vi "Connect and init controller.vi"(7 "axis (0)":u32(ring) items=["1", "2", "3"], 8 "error in (no error)":errorcluster, 9 "Interface types":u32(ring)=1 items=["None", "USB", "TCP", "All"], 10 "path to LUT":path, 11 "path to dll":path) -> (0 "error out":errorcluster, 2 "Rotator":T1={"Controller info"={"deviceNumber"=0, "DeviceType"=3, "ID"=0, "Serial"="", "Address"="", "connected"=FALSE}, "Handle"=0, "FW-Version"=0, "Features"=0, "ActuatorType"=0, "ActuatorName"="", "Axis info"={"Axis status"={"connected"=FALSE, "enabled"=FALSE, "moving"=FALSE, "target"=FALSE, "EotFwd"=FALSE, "EotBwd"=FALSE, "error"=FALSE}, "Position [°]"=0.0, "Freque [Hz]"=0.0, "Voltage [V]"=0.0}, "Capacitance[uF]"=0.0, "Path to DLL"=path ""} {"ActuatorType" items=["Linear", "Rotator", "Goniometer"]; "Controller info"."DeviceType" items=["ANC350res", "ANC350num", "ANC350fps", "No device / invalid"]; "Controller info"."ID" format="%x"})   [LabVIEW 2024, in "SampleRotator.lvlib"]
doc: "Searches for ANC350 devices connected by USB. Connects to first one and reads its info.\n\ninputs:\nPath to DLL; error cluster.\n\noutputs:\nANC350_handle; Controller info; number of found devices; error cluster."
uses:
  SampleRotator.lvlib
  ctl/Rotator all.ctl
  ctl/Axis status.ctl
  <vilib>/Utility/error.llb/Error Cluster From Error Code.vi
  <vilib>/ErrorRing/Error Ring.xnode
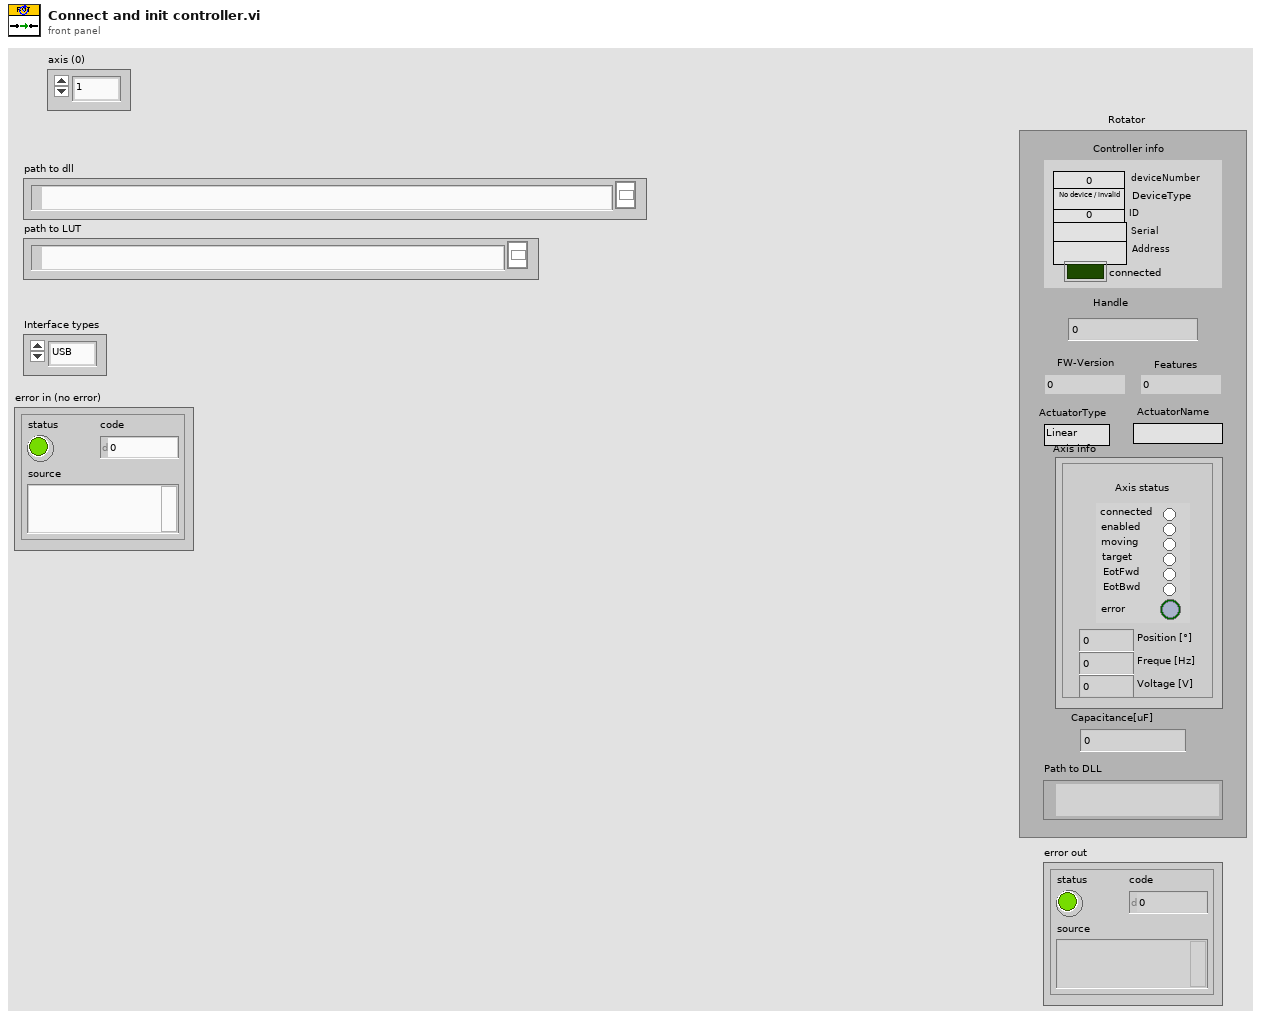
[diagram p1: front panel]
types:
  T1 = typedef "SampleRotator.lvlib/Rotator all.ctl" = cluster{"Controller info":cluster{"deviceNumber":i32, "DeviceType":i32, "ID":u32, "Serial":string, "Address":string, "connected":bool}, "Handle":u64, "FW-Version":i32, "Features":u32, "ActuatorType":u16, "ActuatorName":string, "Axis info":T2, "Capacitance[uF]":dbl, "Path to DLL":path}
  T2 = typedef "SampleRotator.lvlib/Axis status.ctl" = cluster{"Axis status":cluster{"connected":bool, "enabled":bool, "moving":bool, "target":bool, "EotFwd":bool, "EotBwd":bool, "error":bool}, "Position [°]":dbl, "Freque [Hz]":dbl, "Voltage [V]":dbl}
  T3 = cluster{"deviceNumber":i32, "DeviceType":i32, "ID":u32, "Serial":string, "Address":string, "connected":bool}
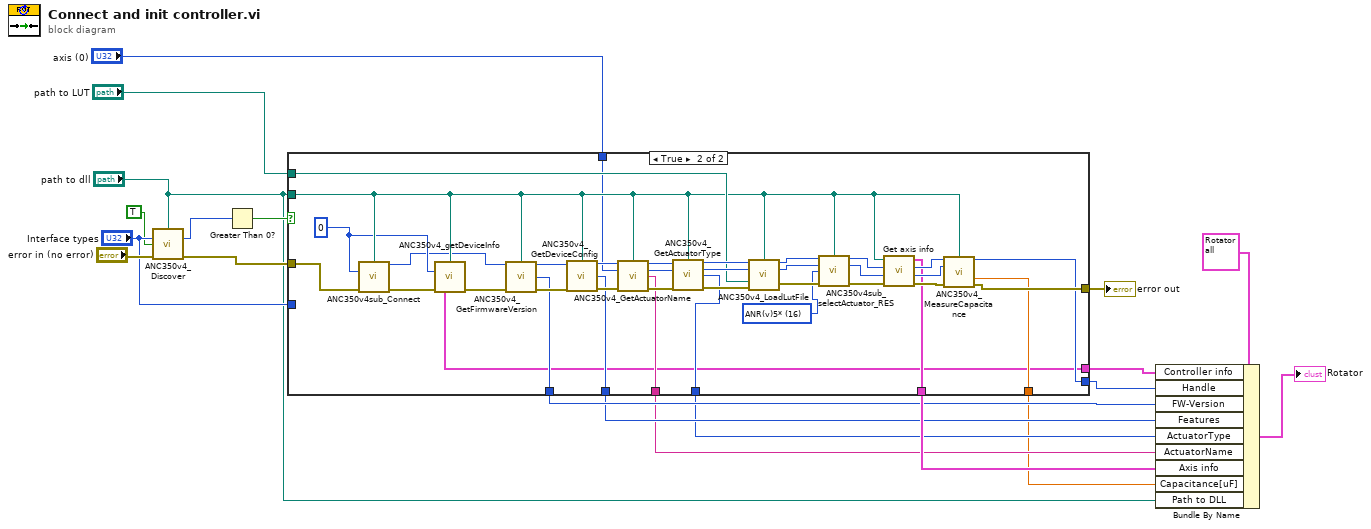
[diagram p0: block diagram]
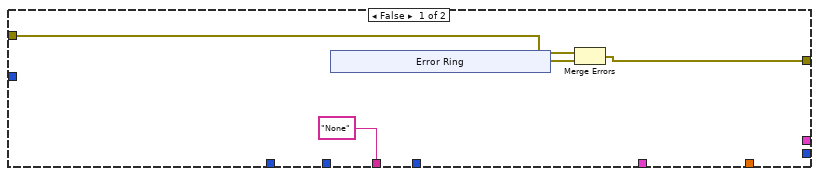
[diagram p2: hidden frame]
diagram:
  n1 = call <instrlib>:"ANC350v4_Discover.vi"("Path to *.DLL"="path to dll", "Interface types"="Interface types", "Load Library (T)\nUnload (F)"=TRUE ("Load Library (T)\nUnload (F)"), "error in"="error in (no error)") -> ("ANC350v4 found"=w16:u32, "error ANC350v4_discover"=w18:errorcluster)  [unwired: 10 in]
  n2 = Greater Than 0?(x=w16) -> (x > 0?=w17:bool)
  n3 = case shown="True" w17 {
    tunnel: "path to dll" -> [_ w33]
    tunnel: "Interface types" -> [_ _]
    tunnel: w18 -> [w22 w30]
    tunnel: [_ w34] -> w11
    tunnel: [w23 w44] -> w15
    tunnel: "path to LUT" -> [_ w57]
    tunnel: [_ w43] -> w10
    tunnel: [_ w42] -> w9
    tunnel: [_ w41] -> w8
    tunnel: [_ w40] -> w7
    tunnel: [_ w39] -> w6
    tunnel: ["None" ("ActuatorName") w38] -> w5
    tunnel: [_ w37] -> w4
    tunnel: "axis (0)" -> [_ w32]
    frame False {
      n4 = xnode "Error Ring"() -> ("error out"=w24:errorcluster)
      n5 = Merge Errors(w22, w24) -> (w23:errorcluster)
    }
    frame True {
      w31 = u32 0 ("deviceNumber")
      w53 = u16 16 items=["ANPx51"=0, "ANPz51"=1, "ANPz51ext"=2, "ANPx101"=3, "ANPz101"=4, "ANPz102"=5, "ANPz101ext"=6, "ANPz111(ext)"=7, "ANPx111(ext)"=8, "ANPx121"=9, "ANPx311"=10, "ANPx321"=11, "ANPx341"=12, "ANGt101"=13, "ANGp101"=14, "ANR(v)101"=15, "ANR(v)5*"=16, "ANR(v)200/240"=17, "ANR(v)220"=18, "Please select type"=99] ("RES-Positionierer")
      n6 = call <instrlib>:"ANC350v4sub_Connect.vi"("Path to *.DLL"=w33, "deviceNumber"=w31, "error in"=w30) -> ("ANC350v4_Handle_Out"=w29:u64, "error ANC350v4_Dis/Connect"=w36:errorcluster)  [unwired: 11 in]
      n7 = call <instrlib>:"ANC350v4_getDeviceInfo.vi"("Path to *.DLL"=w33, "deviceNumber"=w31, "error in"=w36) -> ("output cluster"=w34:T3, "Error_ANC350v4_getDeviceInfo"=w35:errorcluster)  [unwired: 5 in, 6 out]
      n8 = call <instrlib>:"ANC350v4_GetFirmwareVersion.vi"("deviceHandle"=w29, "Path to *.DLL"=w33, "error in"=w35) -> ("deviceHandle"=w51:u64, "FW-Version"=w41:i32, "error ANC350v4_getFirmwareVersion"=w52:errorcluster)  [unwired: 10 in]
      n9 = call <instrlib>:"ANC350v4_GetDeviceConfig.vi"("deviceHandle"=w51, "Path to *.DLL"=w33, "error in"=w52) -> ("deviceHandle"=w65:u64, "features"=w40:u32, "Error_ANC350v4_getDeviceConfig"=w64:errorcluster)  [unwired: 9 in, 1 out]
      n10 = call <instrlib>:"ANC350v4_GetActuatorName.vi"("deviceHandle"=w65, "Path to *.DLL"=w33, "axis"=w32, "error in"=w64) -> ("deviceHandle"=w63:u64, "axis"=w62:u32, "ActuatorName"=w38:string, "error ANC350v4_getActuatorName"=w61:errorcluster)  [unwired: 8 in]
      n11 = call <instrlib>:"ANC350v4_GetActuatorType.vi"("deviceHandle"=w63, "Path to *.DLL"=w33, "axis"=w62, "error in"=w61) -> ("deviceHandle"=w60:u64, "axis"=w59:u32, "ActuatorType"=w39:u16, "error ANC350v4_getActuatorType"=w58:errorcluster)  [unwired: 8 in]
      n12 = call <instrlib>:"ANC350v4_LoadLutFile.vi"("deviceHandle"=w60, "Path to *.DLL"=w33, "axis"=w59, "Path to *.LUT"=w57, "error in"=w58) -> ("deviceHandle"=w55:u64, "axis"=w54:u8, "error ANC350v4_loadLUT"=w56:errorcluster)  [unwired: 8 in]
      n13 = call <instrlib>:"ANC350v4sub_selectActuator_RES.vi"("deviceHandle"=w55, "Path to *.DLL"=w33, "axis"=w54, "RES-Positionierer"=w53, "error in"=w56) -> ("deviceHandle"=w47:u64, "axis"=w46:u8, "error ANC350v4_selectActuator"=w45:errorcluster)  [unwired: 8 in]
      n14 = call "Get axis info.vi"("error in"=w45, "axis"=w46, "deviceHandle"=w47, "path in"=w33) -> ("error out"=w48:errorcluster, "axis out"=w49:u8, "deviceHandle out"=w50:u64, "Axis status"=w43:T2)  [unwired: 4 in]
      n15 = call <instrlib>:"ANC350v4_MeasureCapacitance.vi"("deviceHandle"=w50, "Path to *.DLL"=w33, "axis"=w49, "error in"=w48) -> ("deviceHandle"=w42:u64, "Capacitance"=w37:dbl, "error ANC350v4_frequency"=w44:errorcluster)  [unwired: 8 in, 1 out]
    }
  }
  "error out" <- w15
  n16 = Bundle By Name(cluster=T1 {"Controller info"={"deviceNumber"=0, "DeviceType"=0, "ID"=0, "Serial"="", "Address"="", "connected"=FALSE}, "Handle"=0, "FW-Version"=0, "Features"=0, "ActuatorType"=0, "ActuatorName"="", "Axis info"={"Axis status"={"connected"=FALSE, "enabled"=FALSE, "moving"=FALSE, "target"=FALSE, "EotFwd"=FALSE, "EotBwd"=FALSE, "error"=FALSE}, "Position [°]"=0.0, "Freque [Hz]"=0.0, "Voltage [V]"=0.0}, "Capacitance[uF]"=0.0, "Path to DLL"=path ""} ("Rotator"), "Controller info"=w11, "Handle"=w9, "FW-Version"=w8, "Features"=w7, "ActuatorType"=w6, "ActuatorName"=w5, "Axis info"=w10, "Capacitance[uF]"=w4, "Path to DLL"="path to dll") -> (→"Rotator":T1)
